vi "GlobalRECORD.vi"() -> ()   [LabVIEW 2021]
panel:
  out "record":bool
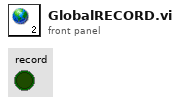
[diagram p1: front panel]
diagram:
